vi "GetClassPath.vi"(8 "error in":errorcluster, 10 "class name":string, 11 "Repository in":refnum<class "NISE_CEF_HierarchyRepo.lvclass">) -> (0 "error out":errorcluster, 2 "class path":path, 3 "Repository out":refnum<class "NISE_CEF_HierarchyRepo.lvclass">)   [LabVIEW 2013, in "NISE_CEF_HierarchyRepo.lvclass"]
doc: "Gets the path to the Class based on the Class Name. \nThe default behavior is build the path of the class on top of the class folder path. The name of the class and the folder it contains needs to be the same. A simple lookup from index and name would be the other option."
uses:
  NISE_CEF_HierarchyRepo.lvclass
  class discovery singleton/class discovery singleton methods.ctl
  class discovery singleton/NISE_CEF_class discovery library.lvlib
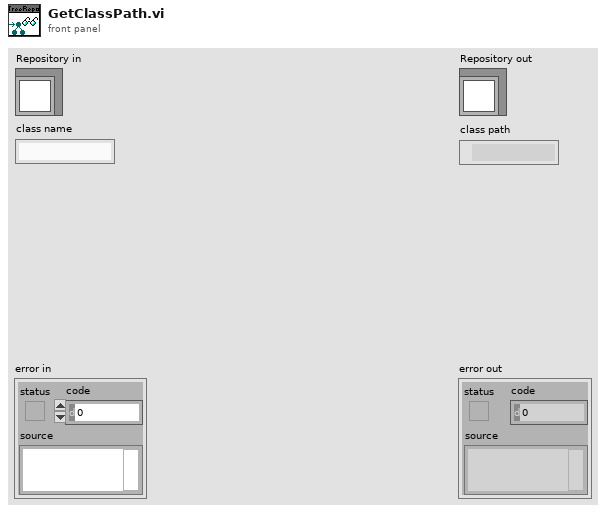
[diagram p1: front panel]
types:
  T1 = typedef "NISE_CEF_class discovery library.lvlib/class discovery singleton methods.ctl" = enum16{"add search paths", "load class by name", "list available classes", "get class path"}
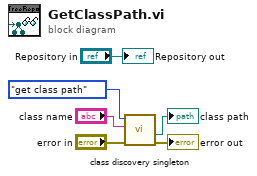
[diagram p0: block diagram]
diagram:
  n1 = call "class discovery singleton.vi"("error in"="error in", "Class Name"="class name", "method"=class_discovery_singleton_methods."get class path") -> ("error out"=→"error out":errorcluster, "class path"=→"class path":path)  [unwired: 5 in, 2 out]
  "Repository out" <- "Repository in"
